vi "Chroma 1905x Series Source Fetch Query.vi"(8 "error in (no error)":errorcluster, 11 "VISA resource name":refnum<visa-resource-name>) -> (0 "error out":errorcluster, 2 "Mode":string, 3 "VISA resource name out":refnum<visa-resource-name>)   [LabVIEW 2025]
doc: "Chroma\n5 Clock Tower Place Suite 210\nMaynard, MA 01754\nTel: 1 800 253-1230\nTel: 1 877 4 A HIPOT\nFax: 1 978-461-4295\nWebsite: www.chroma.com"
panel:
  # "FETCH?"
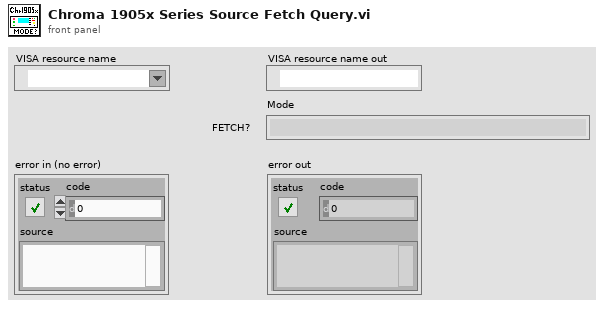
[diagram p1: front panel]
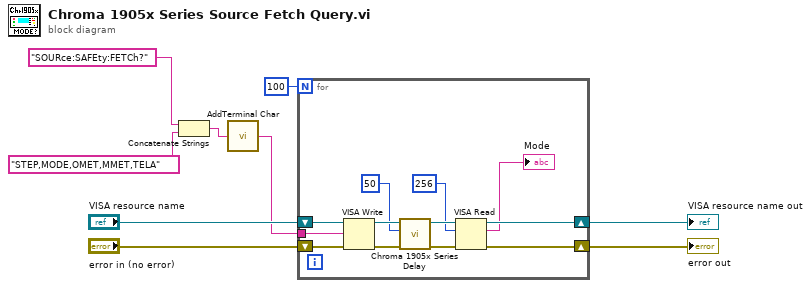
[diagram p0: block diagram]
diagram:
  n1 = Concatenate Strings("SOURce:SAFEty:FETCh?", "STEP,MODE,OMET,MMET,TELA") -> (w2:string)
  n2 = call "AddTerminal Char.vi"("Cmd string"=w2) -> ("Concatenated String"=w7:string)  [unwired: 4 in]
  n3 = for {
    N: 100 -> [_]
    tunnel: w7 -> [w13]
    shift-right: [w11] -> w5
    shift-left: "error in (no error)" -> [w15]
    shift-right: [w12] -> w6
    shift-left: "VISA resource name" -> [w14]
    n4 = VISA Write(VISA resource name=w14, write buffer=w13, error in (no error)=w15) -> (VISA resource name out=w19:refnum<visa-resource-name>, error out=w21:errorcluster)  [unwired: 1 out]
    n5 = call "Chroma 1905x Series Delay.vi"("error in (no error)"=w21, "Time Delay [ms]"=u32 50 ("Time Delay ms"), "VISA resource name"=w19) -> ("error out"=w20:errorcluster, "VISA resource name 2"=w18:refnum<visa-resource-name>)  [unwired: 7 in]
    n6 = VISA Read(VISA resource name=w18, byte count=u32 256, error in (no error)=w20) -> (VISA resource name out=w12:refnum<visa-resource-name>, read buffer=→"Mode":string, error out=w11:errorcluster)  [unwired: 1 out]
  }
  "error out" <- w5
  "VISA resource name out" <- w6
